vi "Stop Command.vi"(8 "error in (no error)":errorcluster, 11 "EL-Go To Height in":refnum<class "EL-Go To Height.lvclass">) -> (0 "error out":errorcluster, 3 "EL-Go To Height out":refnum<class "EL-Go To Height.lvclass">)   [LabVIEW 2014, in "Elevator.lvlib" / "EL-Go To Height.lvlib" / "EL-Go To Height.lvclass"]
uses:
  EL-Go To Height.lvclass
  EL-Go To Height.lvclass/EL-Go To Height.ctl
  Robot Actor Framework/Command Actor/Command Actor Class/Command Actor.lvclass
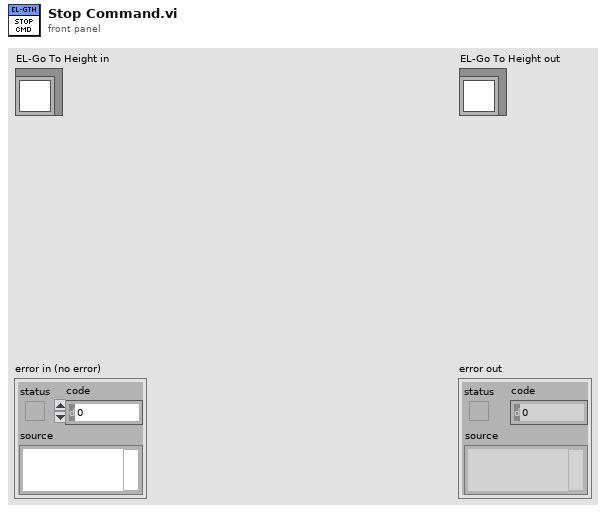
[diagram p1: front panel]
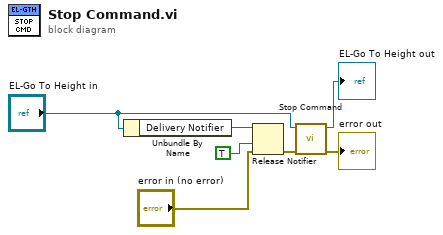
[diagram p0: block diagram]
diagram:
  n1 = Unbundle By Name("EL-Go To Height in") -> ("Delivery Notifier"=w4:refnum<notifier>)
  n2 = Release Notifier(notifier=w4, force destroy? (F)=TRUE, error in (no error)="error in (no error)") -> (error out=w1:errorcluster)  [unwired: 2 out]
  n3 = call-parent "Stop Command.vi"("error in (no error)"=w1, "Command Actor in"="EL-Go To Height in") -> ("error out"=→"error out":errorcluster, "Command Actor out"=→"EL-Go To Height out":refnum<class "EL-Go To Height.lvclass">)  [unwired: 8 in]
